vi "GetFileListing.vi"(10 "patterns":string[](array[string])=["*.py"], 11 "Base Path":path) -> (0 "error out":errorcluster, 1 "Files":path[](array[path]), 3 "Base":path)   [LabVIEW 2022 SP3]
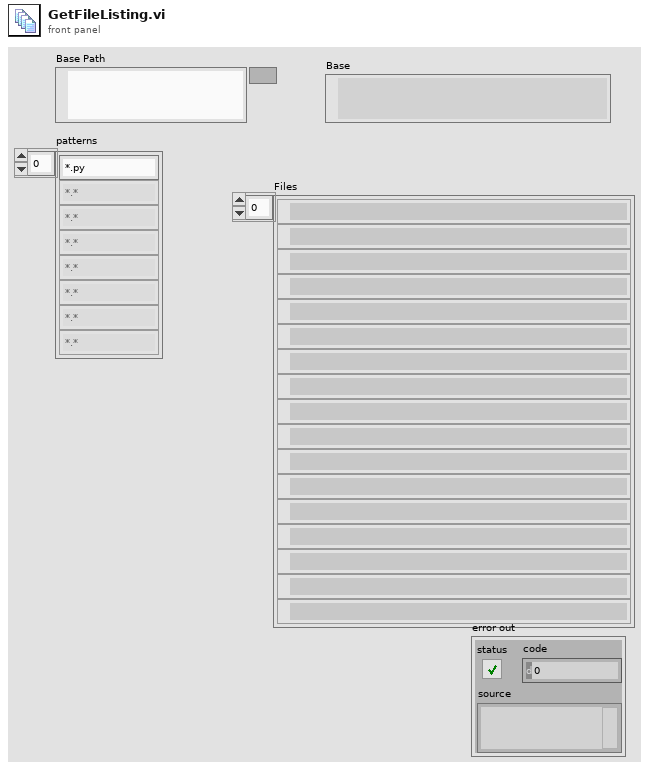
[diagram p1: front panel]
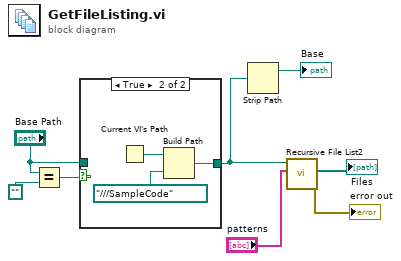
[diagram p0: block diagram]
diagram:
  n1 = Equal?(x="Base Path", y=path "") -> (x = y?=w5:bool)
  n2 = case shown="True" w5 {
    tunnel: [w9 w10] -> w7
    tunnel: "Base Path" -> [w9 _]
    frame False {
    }
    frame True {
      n3 = Current VI's Path() -> (path=w12:path)
      n4 = Build Path(base path=w12, name or relative path=path "../../../SampleCode") -> (appended path=w10:path)
    }
  }
  n5 = Strip Path(path=w7) -> (stripped path=→"Base":path)  [unwired: 1 out]
  n6 = call "Recursive File List2.vi"("patterns"="patterns", "Folder Path"=w7) -> ("error out"=→"error out":errorcluster, "All Files in Dir"=→"Files":path[])  [unwired: 7 in, 1 out]
